vi "fieldMap.vi"() -> (3 "appended array":cluster{"Array":dbl[], "Array 2":dbl[]}[](array[cluster]))   [LabVIEW 2016]
panel:
  in  "Cluster 8":cluster{"Array":dbl[], "Array 2":dbl[]}={"Array"=[5.0, 5.0], "Array 2"=[1.0, 3.4]}
  in  "Cluster 7":cluster{"Array":dbl[], "Array 2":dbl[]}={"Array"=[1.69, 4.39], "Array 2"=[1.2, 1.2]}
  in  "Cluster 6":cluster{"Array":dbl[], "Array 2":dbl[]}={"Array"=[1.0, 1.0], "Array 2"=[0.0, 3.4]}
  in  "Cluster 5":cluster{"Array":dbl[], "Array 2":dbl[]}={"Array"=[0.0, 6.0], "Array 2"=[4.0, 4.0]}
  in  "Cluster 3":cluster{"Array":dbl[], "Array 2":dbl[]}={"Array"=[6.0, 6.0], "Array 2"=[0.0, 4.0]}
  in  "Cluster 2":cluster{"Array":dbl[], "Array 2":dbl[]}={"Array"=[0.0, 6.0], "Array 2"=[0.0, 0.0]}
  in  "Cluster":cluster{"Array":dbl[], "Array 2":dbl[]}={"Array"=[0.0, 0.0], "Array 2"=[0.0, 4.0]}
  out "XY Graph":cluster{dbl[], dbl[]}[](graph)
  in  "Map":cluster{"X\nX":dbl, "Y":dbl}[](array[cluster])=[{"X\nX"=0.0, "Y"=0.0}, {"X\nX"=6.0, "Y"=0.0}, {"X\nX"=6.0, "Y"=4.0}, {"X\nX"=0.0, "Y"=4.0}, {"X\nX"=1.0, "Y"=3.4}, {"X\nX"=1.69, "Y"=1.2}, {"X\nX"=1.0, "Y"=1.2}, {"X\nX"=4.99, "Y"=3.4}, {"X\nX"=4.99, "Y"=4.0}, {"X\nX"=4.99, "Y"=0.0}, {"X\nX"=1.0, "Y"=0.0}, {"X\nX"=1.0, "Y"=4.0}, {"X\nX"=4.99, "Y"=1.2}, {"X\nX"=4.39, "Y"=1.2}, {"X\nX"=4.99, "Y"=1.0}]
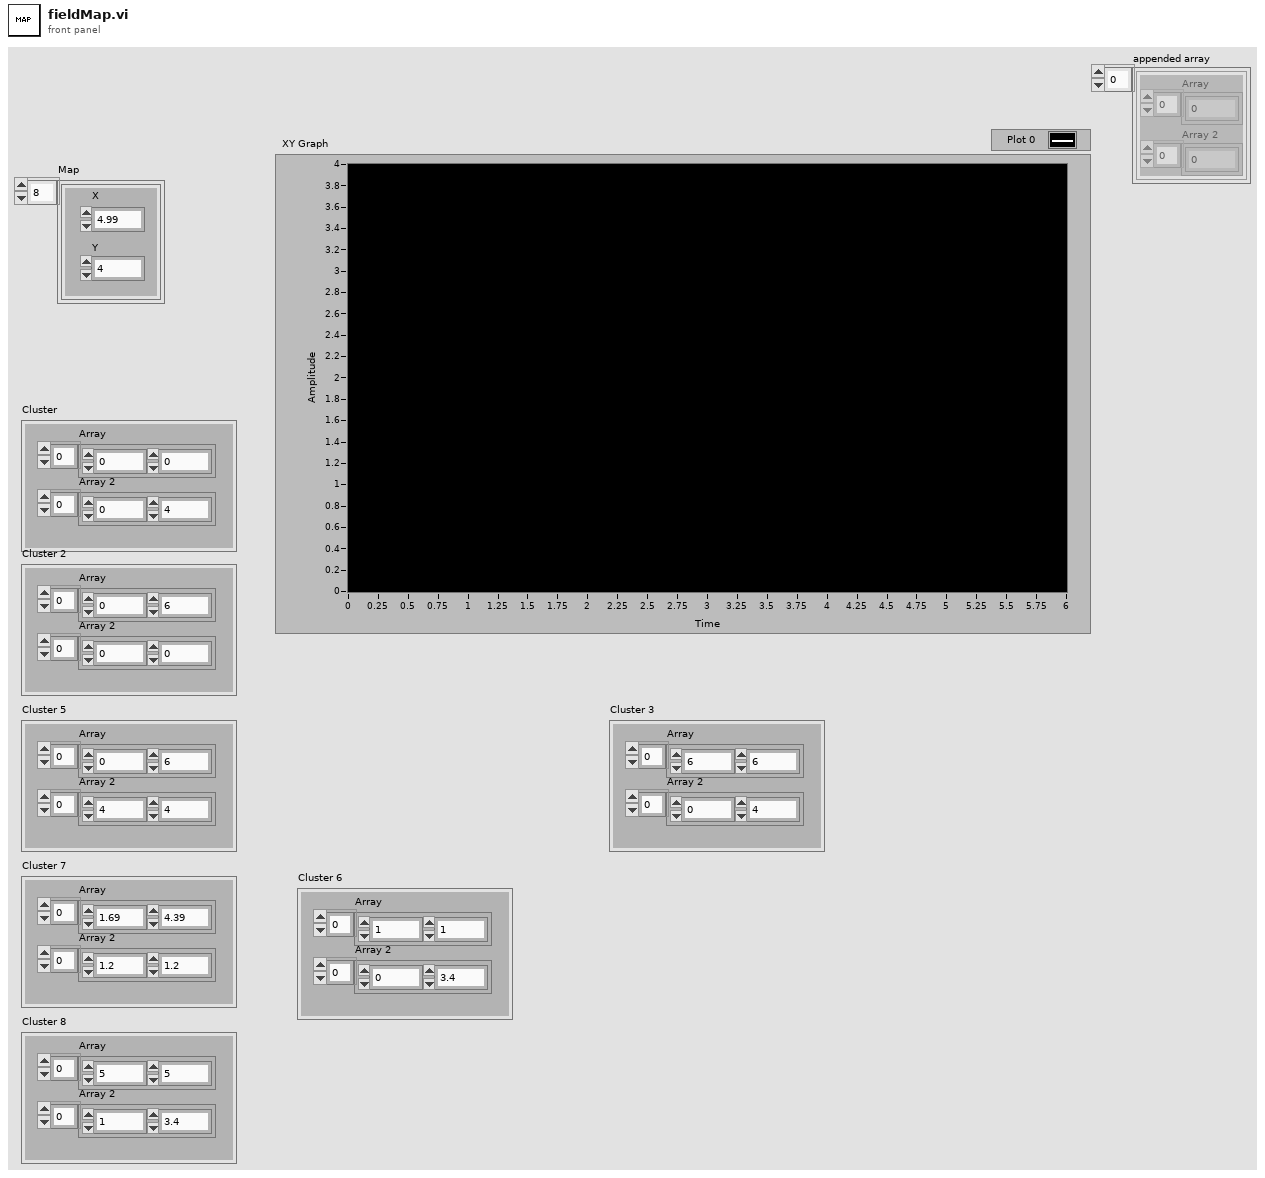
[diagram p1: front panel]
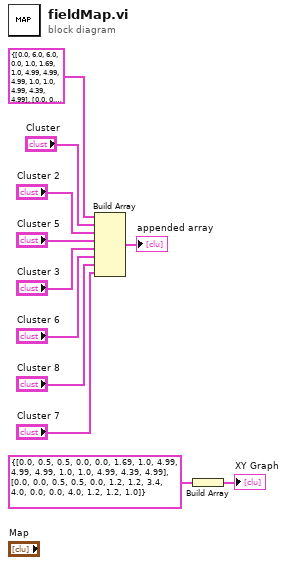
[diagram p0: block diagram]
diagram:
  n1 = Build Array(cluster{dbl[], dbl[]} {[0.0, 6.0, 6.0, 0.0, 1.0, 1.69, 1.0, 4.99, 4.99, 4.99, 1.0, 1.0, 4.99, 4.39, 4.99], [0.0, 0.0, 4.0, 4.0, 3.4, 1.2, 1.2, 3.4, 4.0, 0.0, 0.0, 4.0, 1.2, 1.2, 1.0]} ("output cluster"), "Cluster", "Cluster 2", "Cluster 5", "Cluster 3", "Cluster 6", "Cluster 8", "Cluster 7") -> (→"appended array":cluster{"Array":dbl[], "Array 2":dbl[]}[])
  n2 = Build Array(cluster{dbl[], dbl[]} {[0.0, 0.5, 0.5, 0.0, 0.0, 1.69, 1.0, 4.99, 4.99, 4.99, 1.0, 1.0, 4.99, 4.39, 4.99], [0.0, 0.0, 0.5, 0.5, 0.0, 1.2, 1.2, 3.4, 4.0, 0.0, 0.0, 4.0, 1.2, 1.2, 1.0]} ("output cluster")) -> (→"XY Graph":cluster{dbl[], dbl[]}[])
